vi "Autonomous Independent.vi"() -> ()   [LabVIEW 2012]
doc: "This VI is called when autonomous begins, and will automatically be terminated when autonomous ends. You can carry out timed or sensor driven robot movement independently without needing to return to the caller."
uses:
  Controls/Robot Orientation.ctl
  Autonomous/Autonomous Shooting.vi
  Globals/Autonomous Tipping.vi
  Globals/Robot Build.vi
  Globals/DriveSystemMode.vi
  Globals/Autonomous Joystick Emulation.vi
  Globals/Image Height.vi
  <vilib>/Rock Robotics/WPI/RobotDrive/WPI_RobotDriveArcadeDrive_Standard(NoSaturation).vi
panel:
  in  "Shoot?":bool=TRUE
  in  "Drive to Bridge?":bool=TRUE
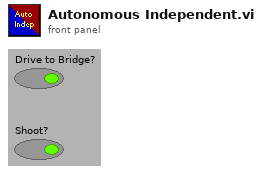
[diagram p1: front panel]
types:
  T1 = typedef "WPI_DigitalInputDevRef.ctl" = cluster{"DevStatus":errorcluster, "DIO Channel":T2, "Digital Module":T3}
  T2 = typedef "FPGA_DIOChannel.ctl" = enum8{"DIO 1", "DIO 2", "DIO 3", "DIO 4", "DIO 5", "DIO 6", "DIO 7", "DIO 8", "DIO 9", "DIO 10", "DIO 11", "DIO 12", "DIO 13", "DIO 14", "Invalid"}
  T3 = typedef "FPGA_TypedefDigitalModule.ctl" = enum16{"Digital Module 1", "Digital Module 2"}
  T4 = typedef "Robot Build.ctl" = enum16{"Practice Bot", "Competition Bot"}
  T5 = typedef "WPI_RobotDriveDevRef.ctl" = cluster{"DevStatus":errorcluster, "Motors[]":T6[], "Square Inputs":bool, "Max Output":dbl, "Isochronous":bool}
  T6 = typedef "WPI_MotorControlDeviceRef.ctl" = cluster{"DeviceStatus":errorcluster, "Type":enum16{"PWM", "CAN"}, "PWM":cluster{"Digital Module":T3, "PWM Channel":T7, "DeadBand":T8}, "CAN":cluster{"Device Number":u8, "Control Mode":T9, "Semaphore":T10, "Max Vout":dbl}, "Invert":bool, "TransformRef":T11, "InvTransformRef":T11}
  T7 = typedef "FPGA_DIOPWMChannel.ctl" = enum8{"PWM 1", "PWM 2", "PWM 3", "PWM 4", "PWM 5", "PWM 6", "PWM 7", "PWM 8", "PWM 9", "PWM 10", "Invalid"}
  T8 = typedef "WPI_PWMDeadband.ctl" = cluster{"Name":string, "maxPositivePwm":i32, "minPositivePwm":i32, "centerPwm":i32, "maxNegativePwm":i32, "minNegativePwm":i32, "angularRange":u16}
  T9 = typedef "WPI_CANJaguar_ControlMode.ctl" = enum8{"Percent VBus", "Current", "Speed", "Position", "Voltage"}
  T10 = typedef "Semaphore RefNum" = refnum<k1>
  T11 = typedef "WPI_PWMTransform_ConPane.ctl" = refnum<vi>
  T12 = typedef "Robot Orientation.ctl" = enum16{"Landscape", "Portrait"}
  T13 = typedef "Drive System Mode.ctl" = enum16{"Normal", "Crab", "Shoot"}
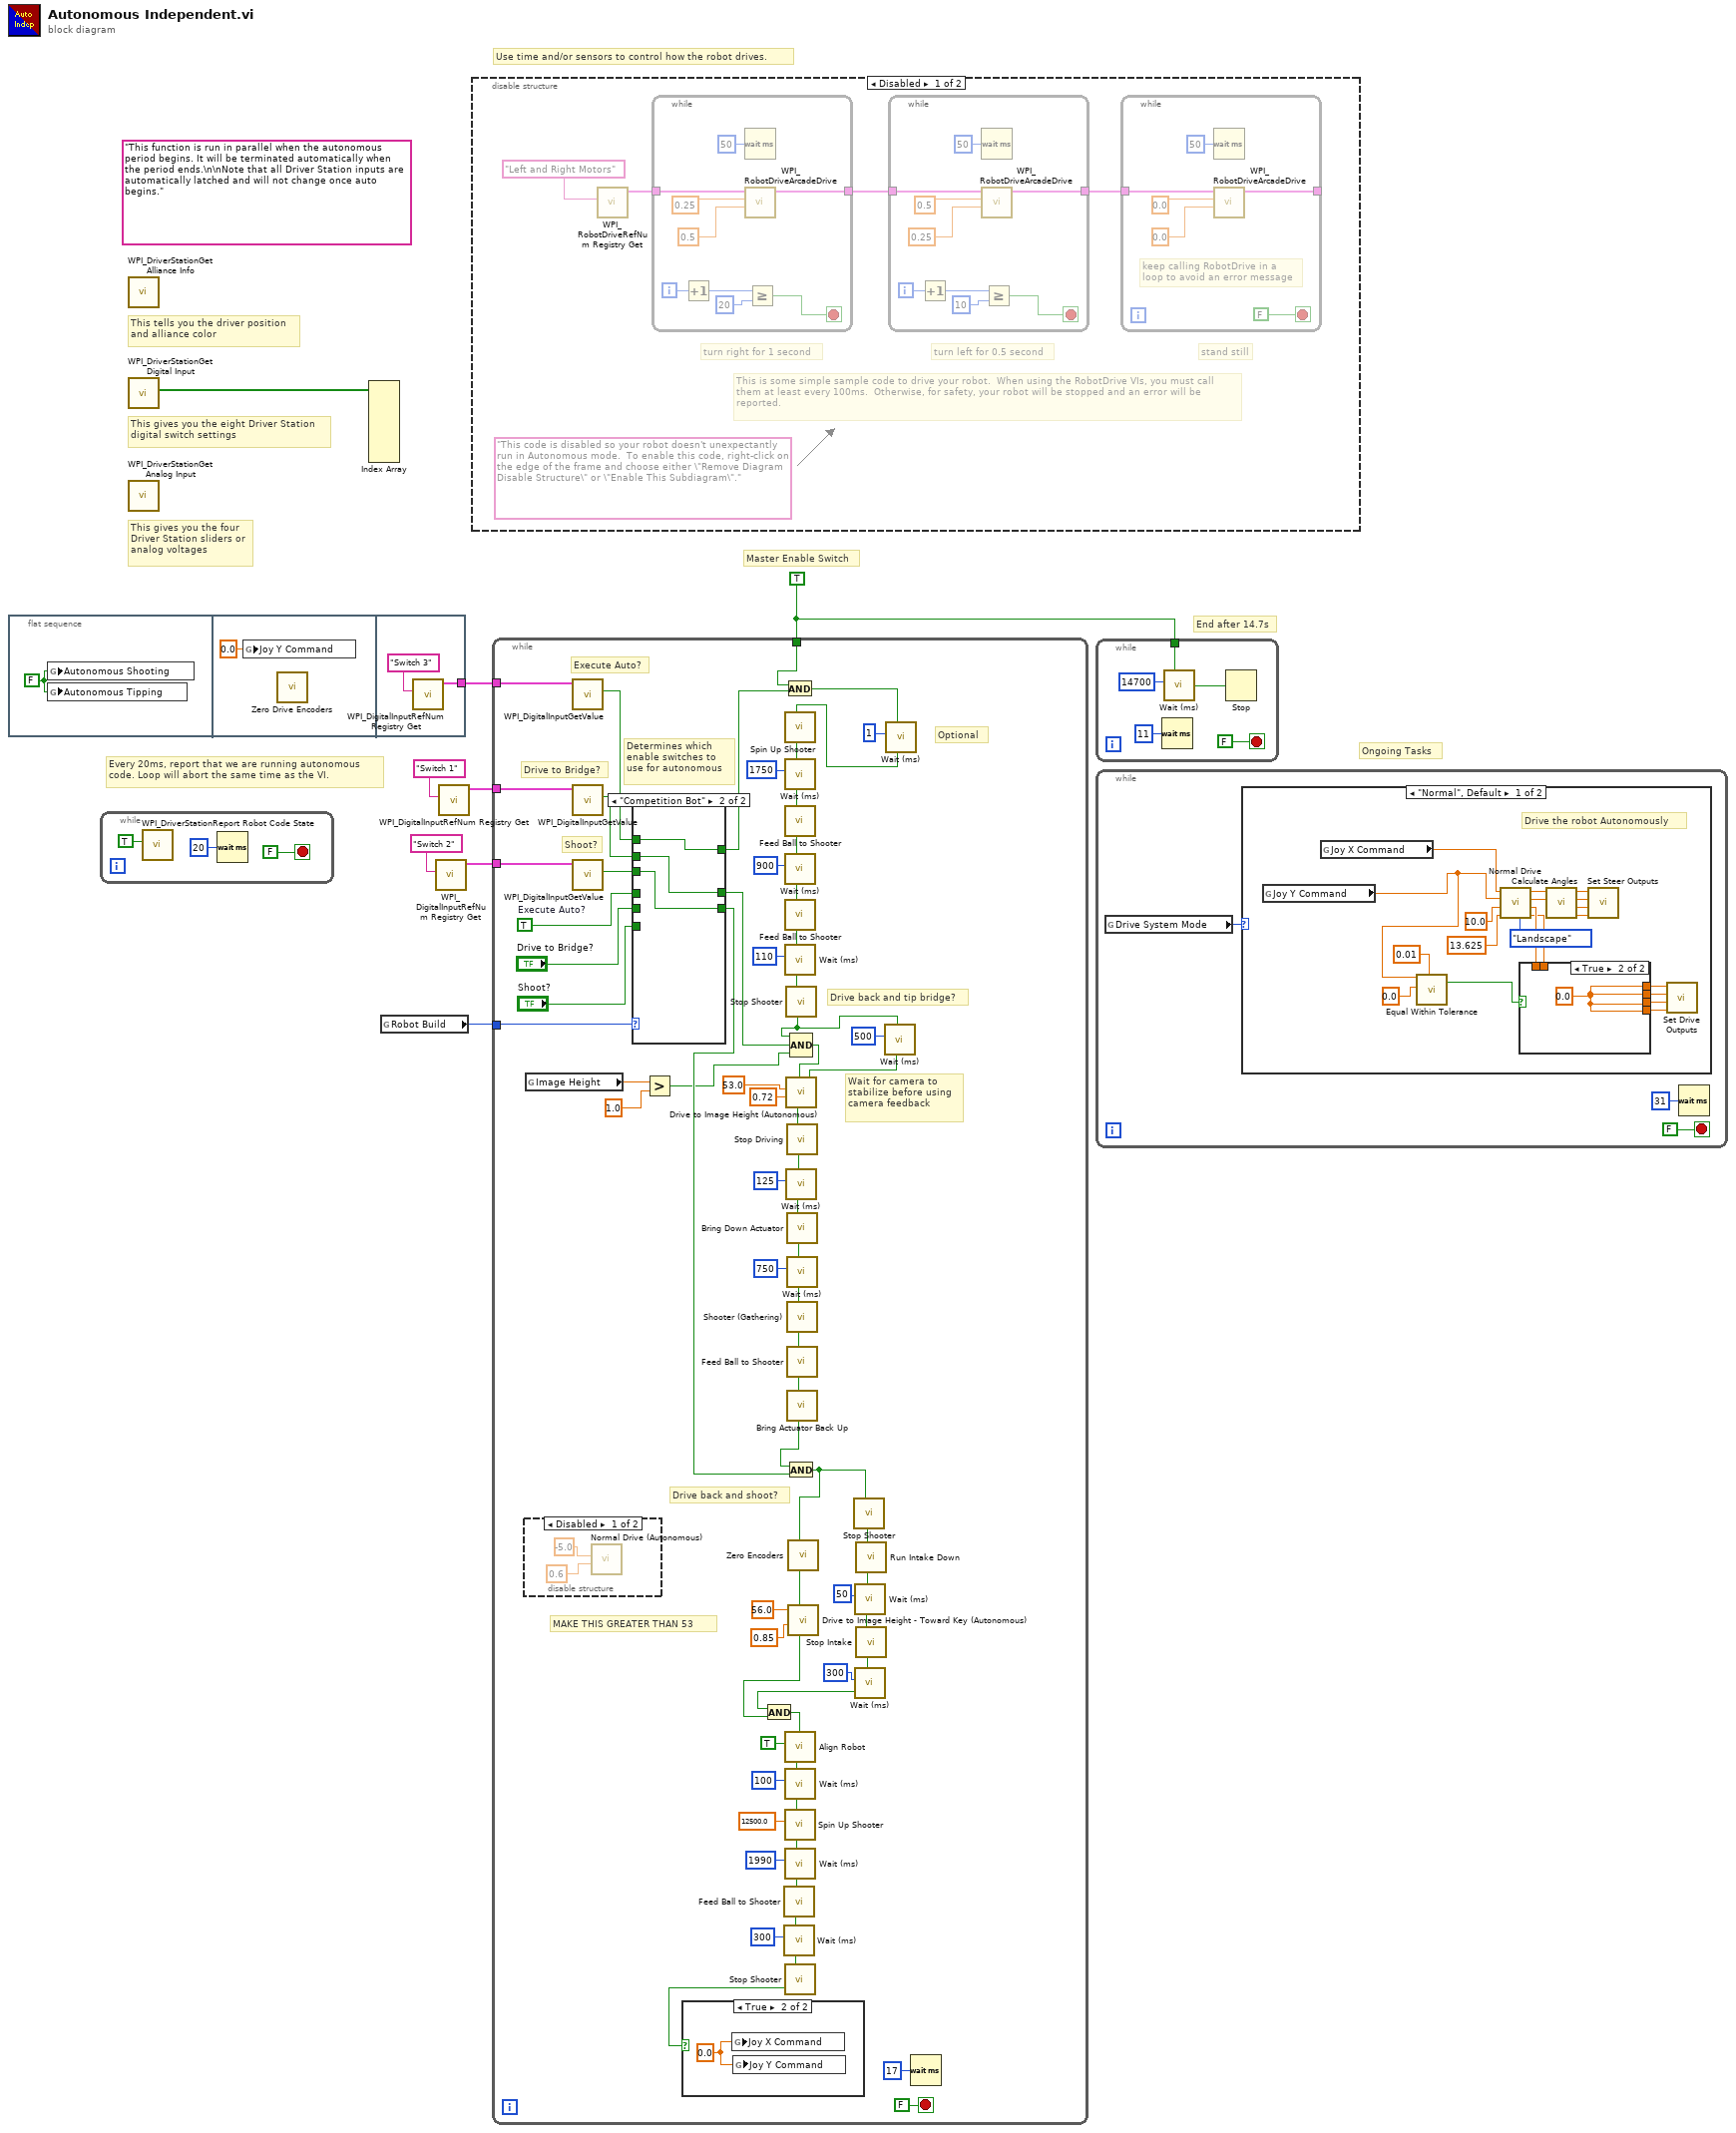
[diagram p0: block diagram]
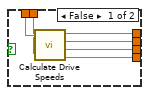
[diagram p2: hidden frame]
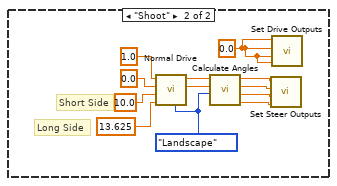
[diagram p3: hidden frame]
diagram:
  w2 = TRUE
  (unwired) "This function is run in parallel when the autonomous period begins. It will be terminated automatically when the period ends.\n\nNote that all Driver Station inputs are automatically latched and will not change once auto begins."
  # "End after 14.7s"
  # "Master Enable Switch"
  # "Ongoing Tasks"
  # "Every 20ms, report that we are running autonomous\ncode. Loop will abort the same time as the VI."
  # "Use time and/or sensors to control how the robot drives."
  # "This tells you the driver position\nand alliance color"
  # "This gives you the eight Driver Station\ndigital switch settings"
  # "This gives you the four\nDriver Station sliders or\nanalog voltages"
  n1 = flat-sequence {
    tunnel: [w11] -> w3
    frame #0 {
      w9 = FALSE ("Autonomous Tipping")
      n2 = global write "Autonomous Shooting.vi" "Autonomous Shooting"(w9) -> ()
      n3 = global write "Autonomous Tipping.vi" "Autonomous Tipping"(w9) -> ()
    }
    frame #1 {
      n4 = global write "Autonomous Joystick Emulation.vi" "Joy Y Command"(0.0 ("Joy Y Command")) -> ()
      n5 = call "Zero Drive Encoders.vi"() -> ()  [unwired: 12 in]
    }
    frame #2 {
      n6 = call <vilib>:"WPI_DigitalInputRefNum Registry Get.vi"("refnum name"="Switch 3") -> ("DigitalInputDevRef"=w11:T1)  [unwired: 9 in, 1 out]
    }
  }
  n7 = while {
    stop <- FALSE stop-if-true
    n8 = call <vilib>:"WPI_DriverStationReport Robot Code State.vi"("Autonomous"=TRUE) -> ()  [unwired: 10 in, 1 out]
    n9 = Wait (ms)(milliseconds to wait=u32 20) -> ()  [unwired: 1 out]
  }
  n10 = call <vilib>:"WPI_DriverStationGet Alliance Info.vi"() -> ()  [unwired: 12 out]
  n11 = call <vilib>:"WPI_DriverStationGet Digital Input.vi"() -> ("Driver Station Digital Input (1-8)"=w8:bool[])  [unwired: 11 out]
  n12 = call <vilib>:"WPI_DriverStationGet Analog Input.vi"() -> ()  [unwired: 12 out]
  n13 = Index Array(array=w8) -> ()  [unwired: 8 in, 8 out]
  n14 = global read "Robot Build.vi" "Robot Build"() -> (w1:T4)
  n15 = call <vilib>:"WPI_DigitalInputRefNum Registry Get.vi"("refnum name"="Switch 2") -> ("DigitalInputDevRef"=w4:T1)  [unwired: 9 in, 1 out]
  n16 = call <vilib>:"WPI_DigitalInputRefNum Registry Get.vi"("refnum name"="Switch 1") -> ("DigitalInputDevRef"=w6:T1)  [unwired: 9 in, 1 out]
  n17 = disable-structure shown="Disabled" {
    frame Disabled {
      (unwired) "This code is disabled so your robot doesn't unexpectantly run in Autonomous mode.  To enable this code, right-click on the edge of the frame and choose either \"Remove Diagram Disable Structure\" or \"Enable This Subdiagram\"."
      # "This is some simple sample code to drive your robot.  When using the RobotDrive VIs, you must call them at least every 100ms.  Otherwise, for safety, your robot will be stopped and an error will be reported."
      # "stand still"
      # "turn left for 0.5 second"
      # "turn right for 1 second"
      n18 = call <vilib>:"WPI_RobotDriveRefNum Registry Get.vi"("refnum name"="Left and Right Motors") -> ("RobotDriveDevRef"=w18:T5)  [unwired: 1 in, 9 out]
      n19 = while {
        tunnel: w18 -> [w43]
        tunnel: [w36] -> w17
        i -> [w39]
        stop <- w37 stop-if-true
        n20 = Increment(x=w39) -> (x+1=w35:i32)
        n21 = Wait (ms)(milliseconds to wait=u32 50) -> ()  [unwired: 1 out]
        n22 = call-poly <vilib>:"WPI_RobotDriveArcadeDrive.vi"("Y axis value"=0.5 ("X axis value"), "X axis value"=0.25, "RobotDriveDevRef"=w43) -> ("RobotDriveDevRef"=w36:T5)  [unwired: 1 in, 7 out]
        n23 = Greater Or Equal?(x=w35, y=20) -> (x >= y?=w37:bool)
      }
      n24 = while {
        tunnel: w17 -> [w34]
        tunnel: [w27] -> w16
        i -> [w30]
        stop <- w28 stop-if-true
        n25 = Increment(x=w30) -> (x+1=w26:i32)
        n26 = Wait (ms)(milliseconds to wait=u32 50) -> ()  [unwired: 1 out]
        n27 = call-poly <vilib>:"WPI_RobotDriveArcadeDrive.vi"("Y axis value"=0.25 ("X axis value"), "X axis value"=0.5, "RobotDriveDevRef"=w34) -> ("RobotDriveDevRef"=w27:T5)  [unwired: 1 in, 7 out]
        n28 = Greater Or Equal?(x=w26, y=10) -> (x >= y?=w28:bool)
      }
      n29 = while {
        tunnel: w16 -> [w25]
        tunnel: [w21] -> _
        stop <- FALSE stop-if-true
        # "keep calling RobotDrive in a loop to avoid an error message"
        n30 = Wait (ms)(milliseconds to wait=u32 50) -> ()  [unwired: 1 out]
        n31 = call-poly <vilib>:"WPI_RobotDriveArcadeDrive.vi"("Y axis value"=0.0 ("X axis value"), "X axis value"=0.0, "RobotDriveDevRef"=w25) -> ("RobotDriveDevRef"=w21:T5)  [unwired: 1 in, 7 out]
      }
    }
    frame Enabled {
    }
  }
  n32 = while {
    tunnel: w2 -> [w69]
    tunnel: w6 -> [w68]
    tunnel: w4 -> [w67]
    tunnel: w3 -> [w66]
    tunnel: w1 -> [w52]
    stop <- FALSE stop-if-true
    w58 = TRUE  # Execute Auto?
    # "MAKE THIS GREATER THAN 53"
    # "Drive back and tip bridge?"
    # "Drive back and shoot?"
    # "Determines which\nenable switches to\nuse for autonomous"
    # "Shoot?"
    # "Drive to Bridge?"
    # "Execute Auto?"
    # "Optional"
    # "Wait for camera to stabilize before using camera feedback"
    n33 = disable-structure shown="Disabled" {
      frame Disabled {
        n34 = call "Normal Drive (Autonomous).vi"("Distance (Feet)"=-5.0, "Percent Speed"=0.6) -> ()  [unwired: 6 in, 1 out]
      }
      frame Enabled {
      }
    }
    n35 = global read "Image Height.vi" "Image Height"() -> (w45:dbl)
    n36 = call <vilib>:"WPI_DigitalInputGetValue.vi"("DigitalInputDevRef"=w66) -> ("Value"=w61:bool)  [unwired: 8 in, 2 out]
    n37 = call <vilib>:"WPI_DigitalInputGetValue.vi"("DigitalInputDevRef"=w68) -> ("Value"=w60:bool)  [unwired: 8 in, 2 out]
    n38 = call <vilib>:"WPI_DigitalInputGetValue.vi"("DigitalInputDevRef"=w67) -> ("Value"=w59:bool)  [unwired: 8 in, 2 out]
    n39 = case shown="\"Competition Bot\"" w52 {
      tunnel: w61 -> [_ w121]
      tunnel: w60 -> [_ w120]
      tunnel: w59 -> [_ w119]
      tunnel: w58 -> [w118 _]
      tunnel: [w117 w120] -> w57
      tunnel: "Drive to Bridge?" -> [w117 _]
      tunnel: [w116 w119] -> w55
      tunnel: [w118 w121] -> w54
      tunnel: "Shoot?" -> [w116 _]
      frame "Practice Bot", Default {
      }
      frame "Competition Bot" {
      }
    }
    n40 = Greater?(x=w45, y=1.0) -> (0:w44:bool)
    n41 = And(x=w69, y=w54) -> (x .and. y?=w63:bool)
    n42 = call "Wait (ms).vi"("Execute"=w63, "milliseconds to wait"=u32 1) -> ("Done Executing"=w64:bool)  [unwired: 6 in]
    n43 = call "Spin Up Shooter.vi"("Execute"=w64) -> ("Done Executing"=w99:bool)  [unwired: 7 in]
    n44 = call "Wait (ms).vi"("Execute"=w99, "milliseconds to wait"=u32 1750) -> ("Done Executing"=w98:bool)  [unwired: 6 in]
    n45 = call "Feed Ball to Shooter.vi"("Execute"=w98) -> ("Done Executing"=w105:bool)  [unwired: 7 in]
    n46 = call "Wait (ms).vi"("Execute"=w105, "milliseconds to wait"=u32 900) -> ("Done Executing"=w103:bool)  [unwired: 6 in]
    n47 = call "Feed Ball to Shooter.vi"("Execute"=w103) -> ("Done Executing"=w104:bool)  [unwired: 7 in]
    n48 = call "Wait (ms).vi"("Execute"=w104, "milliseconds to wait"=u32 110) -> ("Done Executing"=w97:bool)  [unwired: 6 in]
    n49 = call "Stop Shooter.vi"("Execute"=w97) -> ("Done Executing"=w74:bool)  [unwired: 7 in]
    n50 = Compound Arithmetic op=AND(w74, w57, w44) -> (w96:bool)
    n51 = call "Wait (ms).vi"("Execute"=w74, "milliseconds to wait"=u32 500) -> ("Done Executing"=w75:bool)  [unwired: 6 in]
    n52 = call "Drive to Image Height (Autonomous).vi"("Execute"=w96, "Image Height (Pixels)"=53.0, "Percent Velocity"=0.72, "Camera Stabilized?"=w75) -> ("Done Executing"=w108:bool)  [unwired: 4 in]
    n53 = call "Stop Driving.vi"("Execute"=w108) -> ("Done Executing"=w110:bool)  [unwired: 7 in]
    n54 = call "Wait (ms).vi"("Execute"=w110, "milliseconds to wait"=u32 125) -> ("Done Executing"=w109:bool)  [unwired: 6 in]
    n55 = call "Bring Down Actuator.vi"("Execute"=w109) -> ("Done Executing"=w112:bool)  [unwired: 7 in]
    n56 = call "Wait (ms).vi"("Execute"=w112, "milliseconds to wait"=u32 750) -> ("Done Executing"=w79:bool)  [unwired: 6 in]
    n57 = call "Shooter (Gathering).vi"("Execute"=w79) -> ("Done Executing"=w78:bool)  [unwired: 7 in]
    n58 = call "Feed Ball to Shooter.vi"("Execute"=w78) -> ("Done Executing"=w95:bool)  [unwired: 7 in]
    n59 = call "Bring Actuator Back Up.vi"("Execute"=w95) -> ("Done Executing"=w70:bool)  [unwired: 7 in]
    n60 = And(x=w70, y=w55) -> (x .and. y?=w71:bool)
    n61 = call "Zero Encoders.vi"("Execute"=w71) -> ("Done Executing"=w49:bool)  [unwired: 7 in]
    n62 = call "Drive to Image Height - Toward Key (Autonomous).vi"("Execute"=w49, "Image Height (Pixels)"=56.0, "Percent Velocity"=0.85) -> ("Done Executing"=w48:bool)  [unwired: 5 in]
    n63 = call "Stop Shooter.vi"("Execute"=w71) -> ("Done Executing"=w77:bool)  [unwired: 7 in]
    n64 = call "Run Intake Down.vi"("Execute"=w77) -> ("Done Executing"=w92:bool)  [unwired: 7 in]
    n65 = call "Wait (ms).vi"("Execute"=w92, "milliseconds to wait"=u32 50) -> ("Done Executing"=w91:bool)  [unwired: 6 in]
    n66 = call "Stop Intake.vi"("Execute"=w91) -> ("Done Executing"=w90:bool)  [unwired: 7 in]
    n67 = call "Wait (ms).vi"("Execute"=w90, "milliseconds to wait"=u32 300) -> ("Done Executing"=w84:bool)  [unwired: 6 in]
    n68 = And(x=w84, y=w48) -> (x .and. y?=w83:bool)
    n69 = call "Align Robot.vi"("Execute"=w83, "Autonomous Shooting"=TRUE) -> ("Done Executing"=w85:bool)  [unwired: 6 in]
    n70 = call "Wait (ms).vi"("Execute"=w85, "milliseconds to wait"=u32 100) -> ("Done Executing"=w82:bool)  [unwired: 6 in]
    n71 = call "Spin Up Shooter.vi"("Execute"=w82, "Manual Speed"=12500.0) -> ("Done Executing"=w72:bool)  [unwired: 6 in]
    n72 = call "Wait (ms).vi"("Execute"=w72, "milliseconds to wait"=u32 1990) -> ("Done Executing"=w80:bool)  [unwired: 6 in]
    n73 = call "Feed Ball to Shooter.vi"("Execute"=w80) -> ("Done Executing"=w89:bool)  [unwired: 7 in]
    n74 = call "Wait (ms).vi"("Execute"=w89, "milliseconds to wait"=u32 300) -> ("Done Executing"=w87:bool)  [unwired: 6 in]
    n75 = call "Stop Shooter.vi"("Execute"=w87) -> ("Done Executing"=w47:bool)  [unwired: 7 in]
    n76 = case shown="True" w47 {
      frame False {
      }
      frame True {
        w122 = 0.0 ("Joy X Command")
        n77 = global write "Autonomous Joystick Emulation.vi" "Joy X Command"(w122) -> ()
        n78 = global write "Autonomous Joystick Emulation.vi" "Joy Y Command"(w122) -> ()
      }
    }
    n79 = Wait (ms)(milliseconds to wait=u32 17) -> ()  [unwired: 1 out]
  }
  n80 = while {
    tunnel: w2 -> [w127]
    stop <- FALSE stop-if-true
    n81 = Wait (ms)(milliseconds to wait=u32 11) -> ()  [unwired: 1 out]
    n82 = call "Wait (ms).vi"("Execute"=w127, "milliseconds to wait"=u32 14700) -> ("Done Executing"=w128:bool)  [unwired: 6 in]
    n83 = Stop(stop? (T)=w128) -> ()
  }
  n84 = while {
    stop <- FALSE stop-if-true
    n85 = global read "DriveSystemMode.vi" "Drive System Mode"() -> (w130:T13)
    n86 = case shown="\"Normal\", Default" w130 {
      frame "Normal", Default {
        # "Drive the robot Autonomously"
        n87 = global read "Autonomous Joystick Emulation.vi" "Joy Y Command"() -> (w134:dbl)
        n88 = global read "Autonomous Joystick Emulation.vi" "Joy X Command"() -> (w133:dbl)
        n89 = call "Equal Within Tolerance.vi"("Number In"=w134, "Comparison Value"=0.0, "Tolerance"=0.01) -> ("Equality"=w135:bool)  [unwired: 16 in]
        n90 = call "Normal Drive.vi"("Joy X"=w133, "Joy Y"=w134, "Short Radius (Inches)"=10.0 ("Vertical Radius (Inches)"), "Long Radius (Inches)"=13.625 ("Lateral Radius (Inches)"), "Robot Orientation"=Robot_Orientation."Landscape") -> ("Front Left Angle Out"=w144:dbl, "Front Right Angle Out"=w143:dbl, "Left Speed Out"=w142:dbl, "Right Speed Out"=w141:dbl)  [unwired: 1 in]
        n91 = case shown="True" w135 {
          tunnel: [w158 w159] -> w152
          tunnel: [w157 w159] -> w151
          tunnel: [w156 w159] -> w150
          tunnel: [w155 w159] -> w149
          tunnel: w142 -> [w154 _]
          tunnel: w141 -> [w153 _]
          frame False {
            n92 = call "Calculate Drive Speeds.vi"("Left Speed In"=w154, "Right Speed In"=w153) -> ("Front Left Speed"=w158:dbl, "Front Right Speed"=w157:dbl, "Rear Left Speed"=w156:dbl, "Rear Right Speed"=w155:dbl)  [unwired: 2 in]
          }
          frame True {
            w159 = 0.0 ("Front Left Speed")
          }
        }
        n93 = call "Calculate Angles.vi"("Right Angle In"=w143, "Left Angle In"=w144) -> ("Rear Right Steer Out"=w145:dbl, "Rear Left Pot Out"=w146:dbl, "Front Right Pot Out"=w147:dbl, "Front Left Pot Out"=w148:dbl)  [unwired: 2 in]
        n94 = call "Set Steer Outputs.vi"("Rear Right"=w145, "Rear Left"=w146, "Front Right"=w147, "Front Left"=w148) -> ()  [unwired: 8 in]
        n95 = call "Set Drive Outputs.vi"("Rear Right"=w149, "Rear Left"=w150, "Front Right"=w151, "Front Left"=w152) -> ()  [unwired: 8 in]
      }
      frame "Shoot" {
        w164 = 0.0 ("Front Left Speed")
        w165 = Robot_Orientation."Landscape" ("Robot Orientation")
        # "Long Side"
        # "Short Side"
        n96 = call "Normal Drive.vi"("Joy X"=1.0, "Joy Y"=0.0, "Short Radius (Inches)"=10.0 ("Vertical Radius (Inches)"), "Long Radius (Inches)"=13.625 ("Lateral Radius (Inches)"), "Robot Orientation"=w165) -> ("Front Left Angle Out"=w167:dbl, "Front Right Angle Out"=w166:dbl)  [unwired: 1 in, 2 out]
        n97 = call "Calculate Angles.vi"("Robot Orientation"=w165, "Right Angle In"=w166, "Left Angle In"=w167) -> ("Rear Right Steer Out"=w160:dbl, "Rear Left Pot Out"=w161:dbl, "Front Right Pot Out"=w162:dbl, "Front Left Pot Out"=w163:dbl)  [unwired: 1 in]
        n98 = call "Set Steer Outputs.vi"("Rear Right"=w160, "Rear Left"=w161, "Front Right"=w162, "Front Left"=w163) -> ()  [unwired: 8 in]
        n99 = call "Set Drive Outputs.vi"("Rear Right"=w164, "Rear Left"=w164, "Front Right"=w164, "Front Left"=w164) -> ()  [unwired: 8 in]
      }
    }
    n100 = Wait (ms)(milliseconds to wait=u32 31) -> ()  [unwired: 1 out]
  }
